vi "List of Tasks Sent.vi"(8 "error in":errorcluster, 10 "Tasks Standalone":string[][](table)) -> (0 "error out":errorcluster)   [LabVIEW 2020, in "Settings.lvlib"]
doc: "Broadcasts a list of tasks without column names. Acquisition module should decipher the 2D array.\n_____\nCreated using Delacor QMH Event Scripter 6.0.0.121."
uses:
  Settings.lvlib
  List of Tasks Sent Argument--cluster.ctl
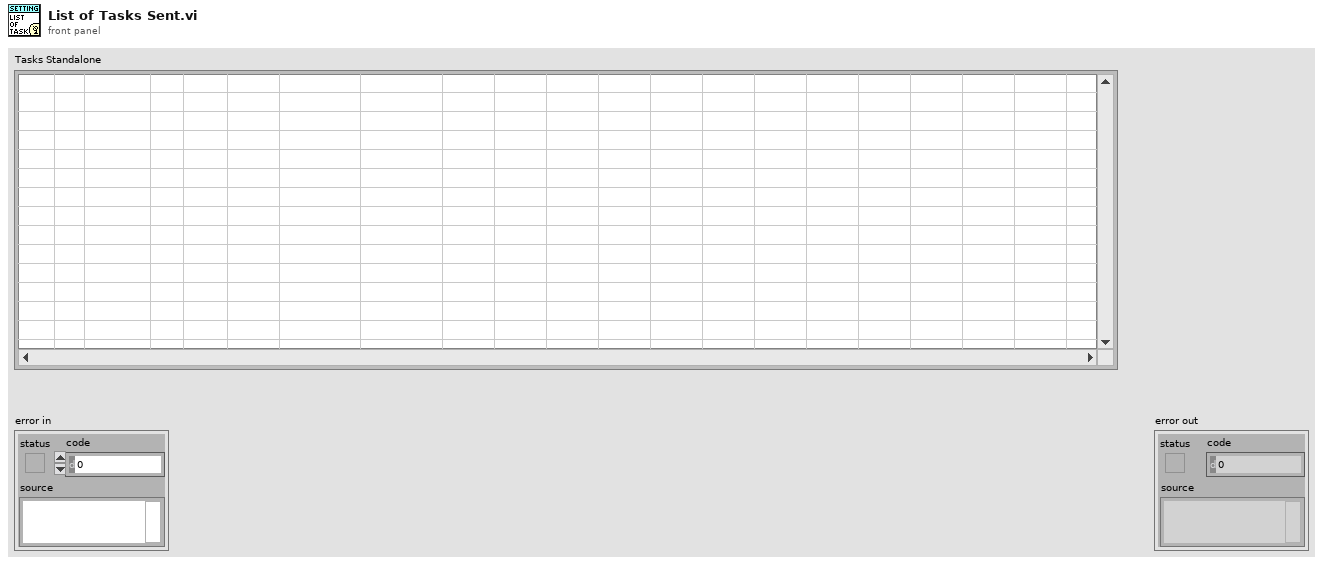
[diagram p1: front panel]
types:
  T1 = typedef "Settings.lvlib/List of Tasks Sent Argument--cluster.ctl" = cluster{"Tasks Standalone":string[][]}
  T2 = typedef "Settings.lvlib/Broadcast Events--cluster.ctl" = cluster{"Module Did Init":refnum<user-event>, "Status Updated":refnum<user-event>, "Error Reported":refnum<user-event>, "Module Did Stop":refnum<user-event>, "Update Module Execution Status":refnum<user-event>, "List of Tasks Sent":refnum<user-event>, "Task Name Set":refnum<user-event>}
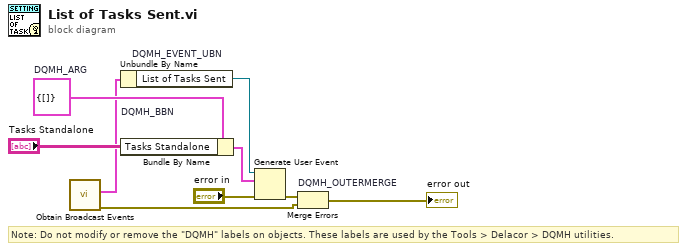
[diagram p0: block diagram]
diagram:
  w4 = T1 {"Tasks Standalone"=[]}  # DQMH_ARG
  # "Note: Do not modify or remove the \"DQMH\" labels on objects. These labels are used by the Tools > Delacor > DQMH utilities."
  n1 = call "Obtain Broadcast Events.vi"() -> ("error out"=w2:errorcluster, "Settings Broadcast Events"=w1:T2)  [unwired: 10 in]
  n2 = Unbundle By Name "DQMH_EVENT_UBN"(w1) -> ("List of Tasks Sent"=w6:refnum<user-event>)
  n3 = Bundle By Name "DQMH_BBN"(cluster=w4, "Tasks Standalone"="Tasks Standalone") -> (w7:T1)
  n4 = Generate User Event(user event=w6, event data cluster=w7, error in="error in") -> (error out=w5:errorcluster)  [unwired: 1 in, 1 out]
  n5 = Merge Errors "DQMH_OUTERMERGE"(w5, w2) -> (→"error out":errorcluster)
